vi "FG Main State.vi"(1 "FG Action":T2, 2 "Main State in":T1=enum."Initialize Sensors") -> (0 "Main State out":T1=enum."Initialize Sensors")   [LabVIEW 2009]
uses:
  Actions for FG's.ctl
  TypeDefs/State Machine/Main State.ctl
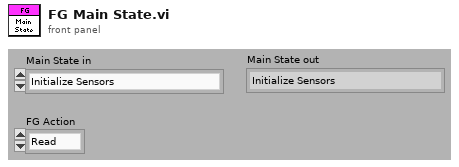
[diagram p1: front panel]
types:
  T1 = typedef "Main State.ctl" = enum16{"Startup", "Wait for Init", "Initialize Sensors", "Wait for Saftey Disable", "Check Saftey", "Wait for GO", "Run", "Remote Control", "Stop"}
  T2 = typedef "Actions for FG's.ctl" = enum16{"Read", "Write"}
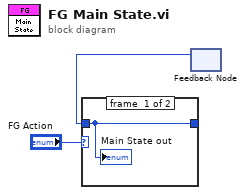
[diagram p0: block diagram]
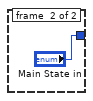
[diagram p2: hidden frame]
diagram:
  n1 = feedback #1() -> (w1:T1)  [unwired: 1 in]
  n2 = case shown="\"Read\", Default" "FG Action" {
    tunnel: [w4 "Main State in"] -> w2
    tunnel: w1 -> [w4 _]
    frame #0 {
      "Main State out" <- w4
    }
    frame #1 {
    }
  }
